vi "LVClass_CameraSet ctor from Copy.vi"(0 "CameraSet (const)":refnum<class "CameraSet.lvclass">, 5 "CameraSet":refnum<class "CameraSet.lvclass">, 11 "error in (no error)":errorcluster) -> (4 "CameraSet (new)":refnum<class "CameraSet.lvclass">, 6 "CameraSet":refnum<class "CameraSet.lvclass">, 15 "error out":errorcluster)   [LabVIEW 2020, in "CameraSet.lvclass"]
doc: "CameraSet constructor.\n\n--------------------------------------------------------------------------------\n\n<B>camera_setIn </B> : Constant Pointer to CameraSet object.\n<B>camera_setOut </B> : Constant Pointer to CameraSet object.\n<B>config_file_path </B> : Absolute path to Haso or Camera configuration file.\n<B>ErrorIn </B> : Error\n<B>ErrorOut </B> : Error\n\n--------------------------------------------------------------------------------"
uses:
  CameraSet.lvclass
  Handle creation.ctl
  CameraSet.lvclass/CameraSet.ctl
  LVClass_CameraSet Read CameraSet.vi
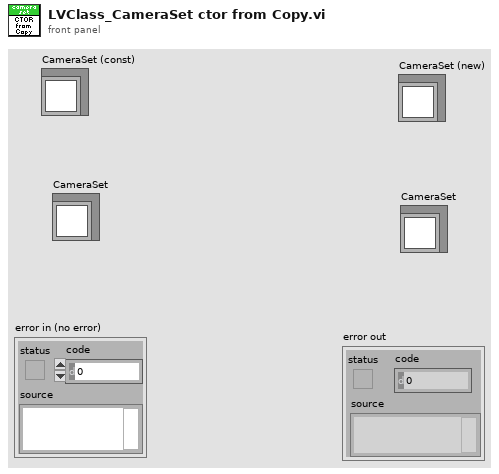
[diagram p1: front panel]
types:
  T1 = typedef "CameraParametersSetup.ctl" = cluster{"Name":string, "Type":T2, "Value":dbl, "BooleanValue":bool, "StringValue":string, "ConnectionParameter":bool}
  T2 = typedef "CameraParameters_Type.ctl" = enum16{"Integer", "Real", "String", "Boolean"}
  T3 = typedef "Handle creation.ctl" = enum16{"By ctor", "By write function"}
  T4 = typedef "ClassID.ctl" = i64
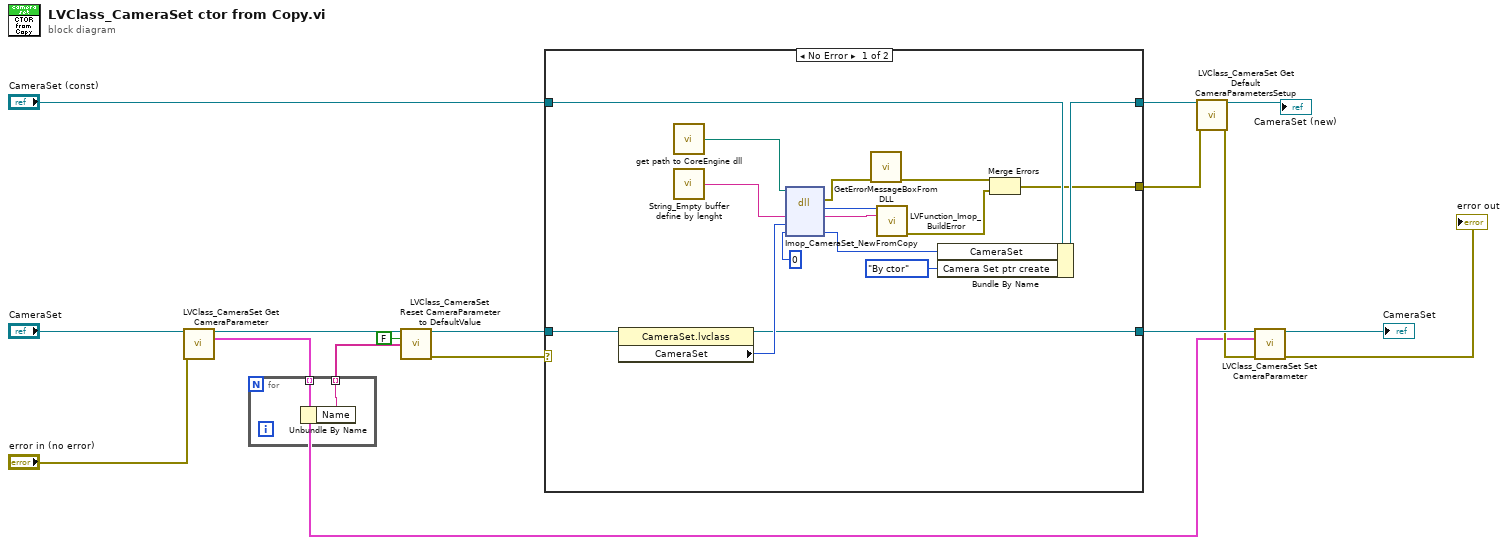
[diagram p0: block diagram]
diagram:
  n1 = call "LVClass_CameraSet Get CameraParameter.vi"("CameraSet in"="CameraSet", "error in (no error)"="error in (no error)") -> ("CameraSet out"=w14:refnum<class "CameraSet.lvclass">, "AllCurrentValueSetAndGet"=w3:T1[])  [unwired: 10 in, 2 out]
  n2 = for {
    tunnel: w3 -> [w18] mode=indexing
    tunnel: [w17] -> w9 mode=indexing
    n3 = Unbundle By Name(w18) -> ("Name"=w17:string)
  }
  n4 = call "LVClass_CameraSet Reset CameraParameter to DefaultValue.vi"("CameraSet out"=w14, "ResetAllParametersToDefault"=FALSE, "ListOfParametersToResetDefault"=w9) -> ("CameraSet out"=w8:refnum<class "CameraSet.lvclass">, "error out"=w1:errorcluster)  [unwired: 11 in]
  n5 = case shown="No Error" w1 {
    selector: w1 -> [_ w36]
    tunnel: w8 -> [w21 w35]
    tunnel: "CameraSet (const)" -> [w29 w37]
    tunnel: [w28 w37] -> w12
    tunnel: [w22 w36] -> w10
    tunnel: [w19 w35] -> w7
    frame No Error {
      n6 = property class="CameraSet.lvclass"(reference=w21) -> (reference out=w19:refnum<class "CameraSet.lvclass">, "CameraSet"=w20:T4)  [unwired: 1 in, 1 out]
      n7 = call "get path to CoreEngine dll.vi"() -> ("path to c_interface_vc100.dll"=w27:path)  [unwired: 12 in, 3 out]
      n8 = call "String_Empty buffer define by lenght.vi"() -> ("Empty buffer"=w34:string)  [unwired: 1 in]
      n9 = dll-call lib="D:/soft/HASO_v3/SVN_trunk/ImOpCoreEngine4_LV2011/DLLs/c_interface_vc100.dll" fn="Imop_CameraSet_NewFromCopy"(path in=w27, "message"=w34, "CameraSet"=w20, "NewCameraSet"=0 ("objet")) -> (error out=w26:errorcluster, "return type"=w31:i32, "message"=w32:string, "NewCameraSet"=w33:i64)  [unwired: 3 in, 1 out]
      n10 = call "GetErrorMessageBoxFromDLL.vi"("error IN"=w26) -> ("error OUT"=w24:errorcluster)  [unwired: 10 in]
      n11 = call "LVFunction_Imop_BuildError.vi"("code"=w31, "String to Prepend to source (\"\")"=w32) -> ("error out"=w23:errorcluster)  [unwired: 13 in]
      n12 = Bundle By Name(cluster=w29, "CameraSet"=w33, "Camera Set ptr create"=Handle_creation."By ctor") -> (w28:refnum<class "CameraSet.lvclass">)
      n13 = Merge Errors(w24, w23) -> (w22:errorcluster)
    }
    frame Error {
    }
  }
  n14 = call "LVClass_CameraSet Get Default CameraParametersSetup.vi"("CameraSet in"=w12, "error in (no error)"=w10) -> ("CameraSet out"=→"CameraSet (new)":refnum<class "CameraSet.lvclass">, "error out"=w4:errorcluster)  [unwired: 9 in, 3 out]
  n15 = call "LVClass_CameraSet Set CameraParameter.vi"("CameraSet out"=w7, "CameraParametersSettable"=w3, "error in (no error)"=w4) -> ("CameraSet out"=→"CameraSet":refnum<class "CameraSet.lvclass">, "error out"=→"error out":errorcluster)  [unwired: 11 in]
